vi "Measurement Logic.vi"(8 "error in":errorcluster, 9 "measurement configuration":T2={"Frequency"=1.2, "Duty Cycle"=32.0, "Number of Pulses"=64, "Counter Resource Name"="Lorem ipsum dolor sit", "Output Resource Name"="/Dev1/PFI12"} {"Number of Pulses" format="%.6f"; "Duty Cycle" format="%.6f"; "Frequency" format="%.6f"}, 10 "measure call context in":refnum<class "Measure Call Context.lvclass">) -> (0 "error out":errorcluster, 1 "measurement results":T1, 2 "measure call context out":refnum<class "Measure Call Context.lvclass">)   [LabVIEW 2025, in "WorkflowDO.lvclass"]
doc: "Contains the core logic for executing the measurement."
uses:
  WorkflowDO.lvclass
  <vilib>/Plug-In SDKs/Measurements/Measure Call Context/Measure Call Context.lvclass
  Measurement Configuration.ctl
  Measurement Results.ctl
  <vilib>/DAQmx/create/channels.llb/DAQmx Create Channel (CO-Pulse Generation-Frequency).vi
  <vilib>/DAQmx/configure/timing.llb/DAQmx Timing (Implicit).vi
  <extravilib>/ChannelInstances/Event Messenger-bool/Instantiate.vi
  WorkflowDO.lvclass/WorkflowDO.ctl
  <resource>/objmgr/daqmx.rc
panel:
  out "Actual Duty Cycle":dbl
  out "Actual Frequency":dbl
  in  "Stop":bool
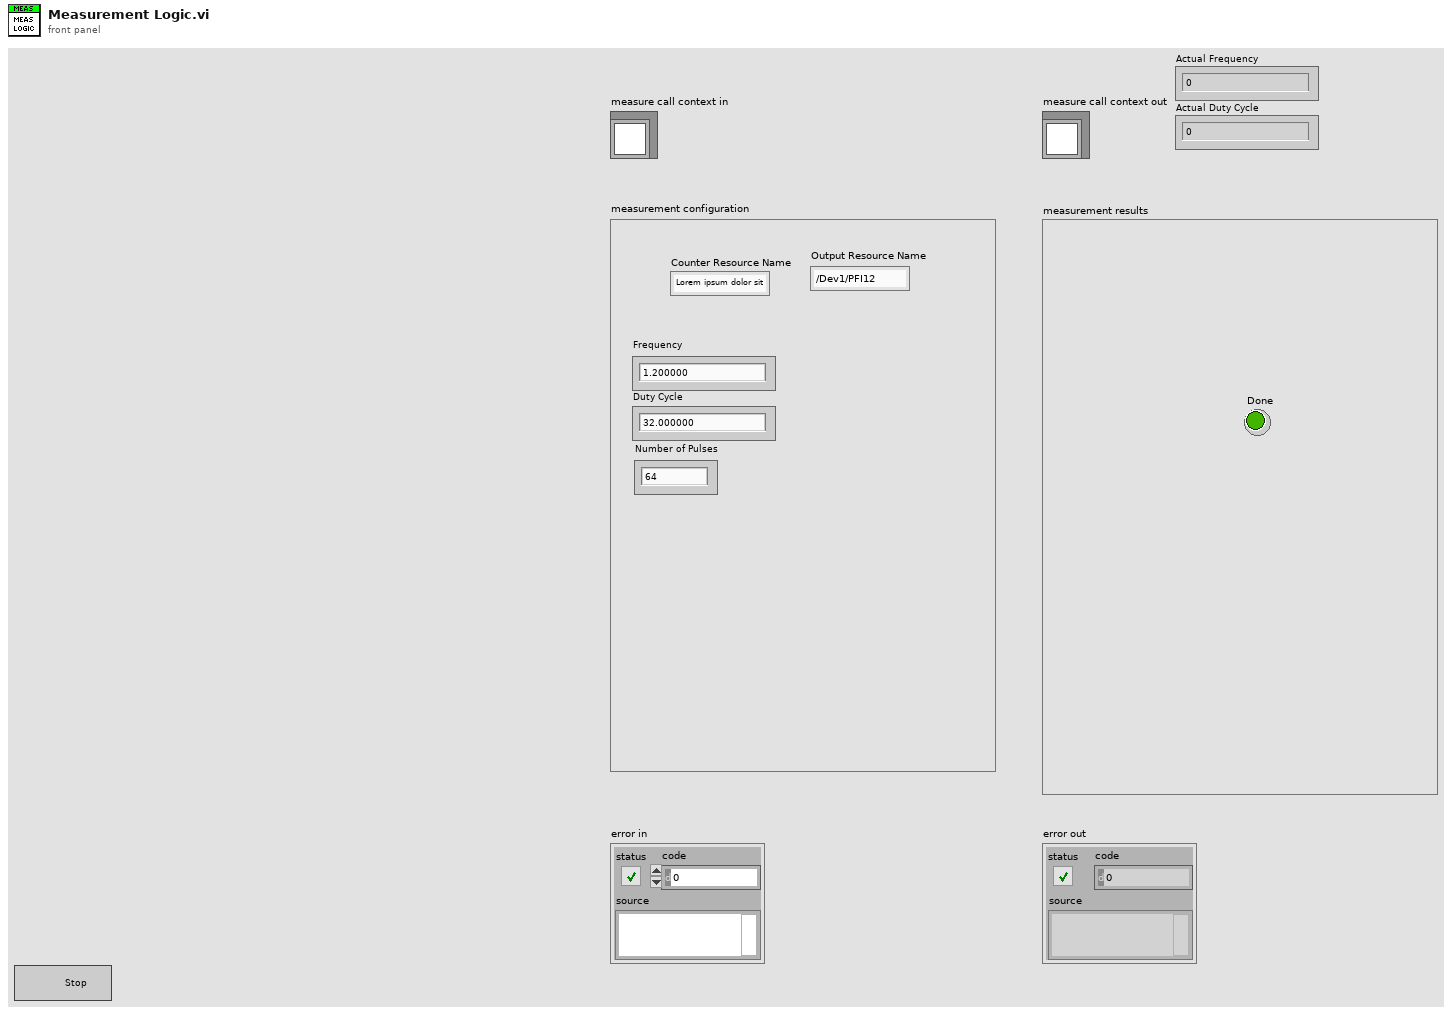
[diagram p1: front panel]
types:
  T1 = typedef "WorkflowDO.lvclass/Measurement Results.ctl" = cluster{"Done":bool}
  T2 = typedef "WorkflowDO.lvclass/Measurement Configuration.ctl" = cluster{"Frequency":dbl, "Duty Cycle":dbl, "Number of Pulses":i32, "Counter Resource Name":string, "Output Resource Name":string}
  T3 = typedef "Event Messenger-bool.lvlib/))Channel.ctl" = refnum<queue>
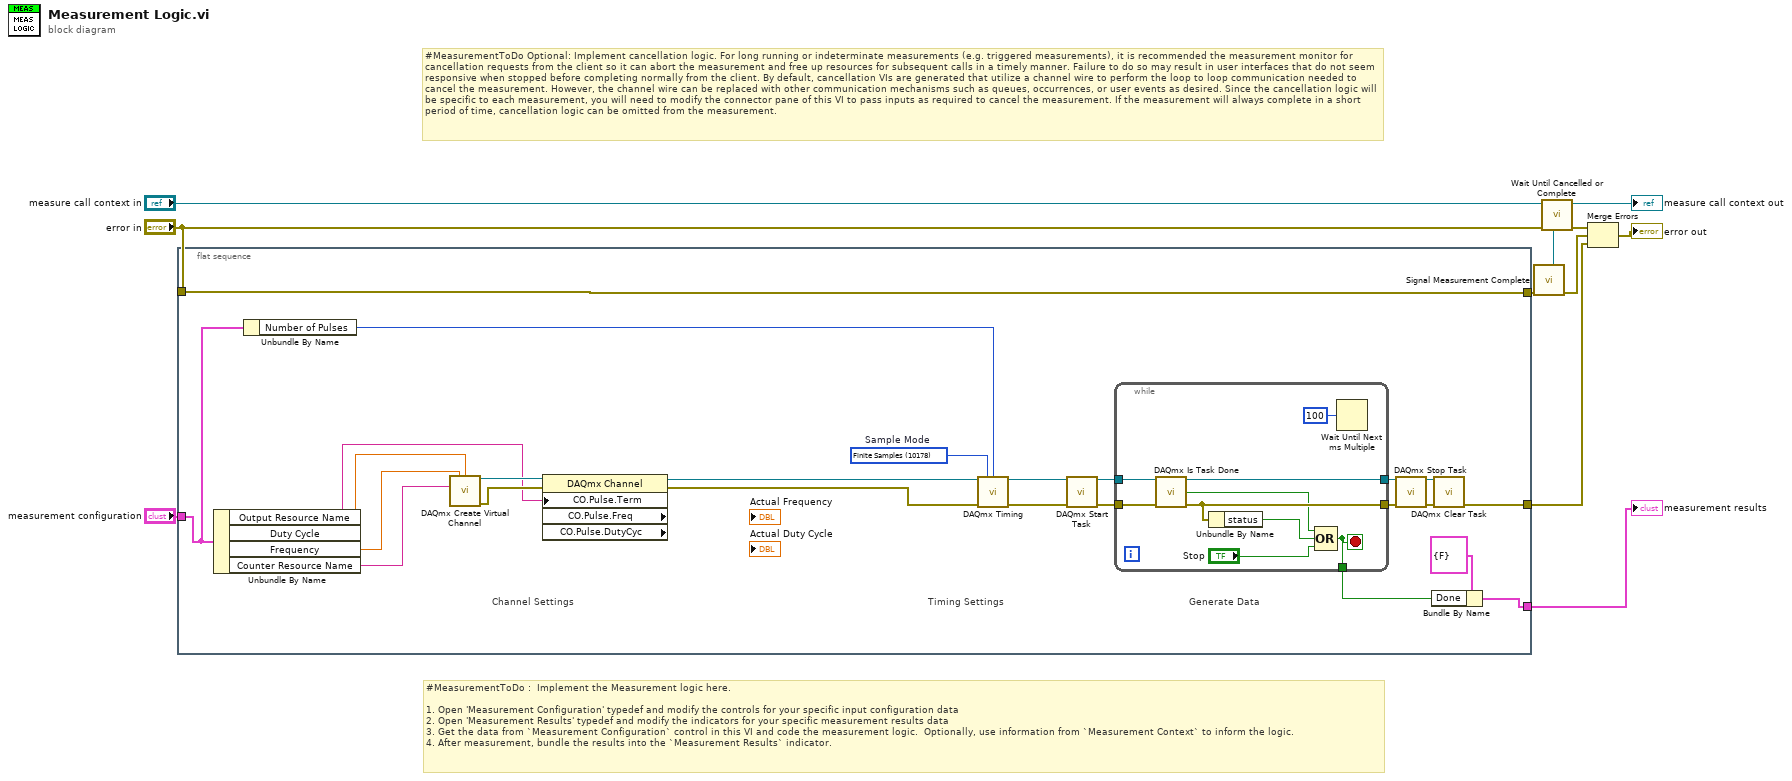
[diagram p0: block diagram]
diagram:
  # "#MeasurementToDo Optional: Implement cancellation logic. For long running or indeterminate measurements (e.g. triggered measurements), it is recommended the measurement monitor for cancellation requests from the client so it can abort the measurement and free up resources for subsequent calls in a timely manner. Failure to do so may result in user interfaces that do not seem responsive when stopped before completing normally from the client. By default, cancellation VIs are generated that utilize a channel wire to perform the loop to loop communication needed to cancel the measurement. However, the channel wire can be replaced with other communication mechanisms such as queues, occurrences, or user events as desired. Since the cancellation logic will be specific to each measurement, you will need to modify the connector pane of this VI to pass inputs as required to cancel the measurement. If the measurement will always complete in a short period of time, cancellation logic can be omitted from the measurement."
  # "#MeasurementToDo :  Implement the Measurement logic here.\n\n1. Open 'Measurement Configuration' typedef and modify the controls for your specific input configuration data\n2. Open 'Measurement Results' typedef and modify the indicators for your specific measurement results data\n3. Get the data from `Measurement Configuration` control in this VI and code the measurement logic.  Optionally, use information from `Measurement Context` to inform the logic.\n4. After measurement, bundle the results into the `Measurement Results` indicator."
  n1 = flat-sequence {
    tunnel: "measurement configuration" -> [w16]
    tunnel: "error in" -> [w35]
    tunnel: [w35] -> w7
    tunnel: [w21] -> w2
    tunnel: [w14] -> w1
    frame #0 {
      w34 = 10178 items=["Finite Samples"=10178, "Continuous Samples"=10123, "Hardware Timed Single Point"=12522]  # Sample Mode
      # "Generate Data"
      # "Timing Settings"
      # "Channel Settings"
      n2 = Unbundle By Name(w16) -> ("Output Resource Name"=w20:string, "Duty Cycle"=w19:dbl, "Frequency"=w18:dbl, "Counter Resource Name"=w17:string)
      n3 = Unbundle By Name(w16) -> ("Number of Pulses"=w15:i32)
      n4 = call-poly <vilib>:"DAQmx Create Virtual Channel.vi"("frequency"=w18, "duty cycle"=w19, "counter"=w17) -> ("task out"=w29:refnum<k21>, "error out"=w28:errorcluster)  [unwired: 11 in]
      n5 = property class="DAQmx Channel" props=["CO.Pulse.Term", "CO.Pulse.Freq", "CO.Pulse.DutyCyc"](reference=w29, error in=w28, "CO.Pulse.Term"=w20) -> (reference out=w26:refnum<k21>, error out=w27:errorcluster)  [unwired: 2 out]
      n6 = call-poly <vilib>:"DAQmx Timing.vi"("task/channels in"=w26, "sample mode"=w34, "samples per channel"=w15, "error in"=w27) -> ("task out"=w31:refnum<k21>, "error out"=w30:errorcluster)  [unwired: 10 in]
      n7 = call <vilib>:"DAQmx Start Task.vi"("task/channels in"=w31, "error in"=w30) -> ("task out"=w33:refnum<k21>, "error out"=w32:errorcluster)  [unwired: 12 in]
      n8 = while {
        tunnel: w33 -> [w44]
        tunnel: w32 -> [w43]
        tunnel: [w41] -> w22
        tunnel: [w42] -> w23
        tunnel: [w36] -> w12
        stop <- w36 stop-if-true
        n9 = call <vilib>:"DAQmx Is Task Done.vi"("task/channels in"=w44, "error in"=w43) -> ("task out"=w42:refnum<k21>, "task done?"=w37:bool, "error out"=w41:errorcluster)  [unwired: 11 in]
        n10 = Unbundle By Name(w41) -> ("status"=w40:bool)
        n11 = Compound Arithmetic op=OR(w37, w40, "Stop") -> (w36:bool)
        n12 = Wait Until Next ms Multiple(millisecond multiple=u32 100) -> ()  [unwired: 1 out]
      }
      n13 = call <vilib>:"DAQmx Stop Task.vi"("task/channels in"=w23, "error in"=w22) -> ("task out"=w25:refnum<k21>, "error out"=w24:errorcluster)  [unwired: 12 in]
      n14 = Bundle By Name(cluster=T1 {"Done"=FALSE} ("measurement results"), "Done"=w12) -> (w14:T1)
      n15 = call <vilib>:"DAQmx Clear Task.vi"("task in"=w25, "error in"=w24) -> ("error out"=w21:errorcluster)  [unwired: 13 in]
    }
  }
  n16 = call "Signal Measurement Complete.vi"("error in (no error)"=w7) -> ("error out"=w5:errorcluster, "done channel"=w6:T3)  [unwired: 9 in]
  n17 = call "Wait Until Cancelled or Complete.vi"("done channel"=w6, "error in (no error)"="error in", "measure call context in"="measure call context in") -> ("error out"=w4:errorcluster, "measure call context out"=→"measure call context out":refnum<class "Measure Call Context.lvclass">)  [unwired: 7 in]
  n18 = Merge Errors(w4, w5, w2) -> (→"error out":errorcluster)
  "measurement results" <- w1
